vi "getLockStatus.vi"(8 "error":errorcluster, 11 "connection ID":refnum<k5>) -> (0 "error out":errorcluster, 1 "authorized":bool, 2 "locked":bool, 3 "connection ID out":refnum<k5>)   [LabVIEW 2016, in "sen_api.lvlib"]
doc: "This function returns if the device is locked and if the current client is authorized to use the device."
uses:
  sen_api.lvlib
panel:
  out "jsonRespIn":string
  out "JSON-response":string="{\"jsonrpc\":\"2.0\",\"method\":\"\",\"params\":[5,1.245,true,\"name\"],\"id\":\"1\"}"
  out "JSON request":string
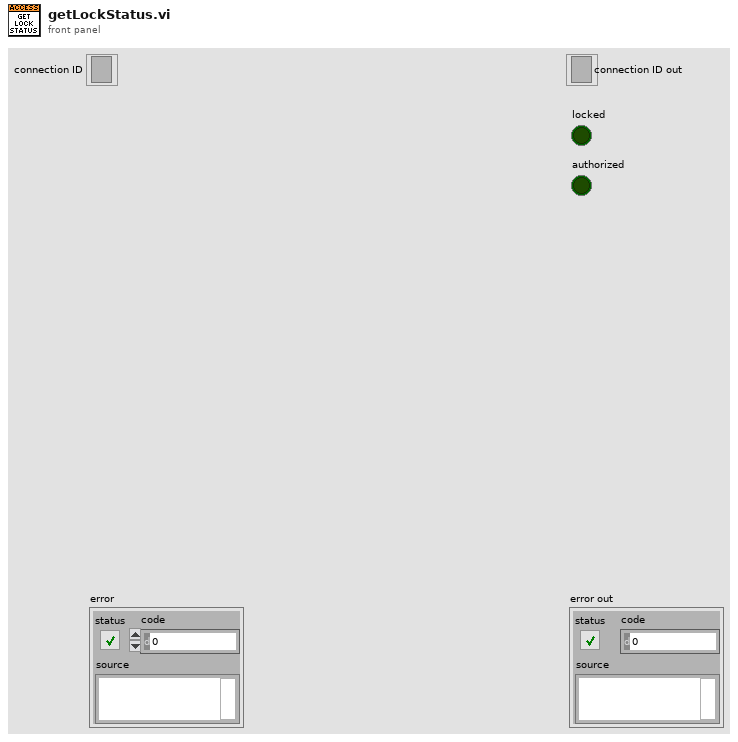
[diagram p1: front panel]
types:
  T1 = cluster{"jsonrpc":string, "method":string, "params":string[], "id":string, "api":i32, "pid":string}
  T2 = enum16{"Standard", "Buffered", "CRLF", "Immediate"}
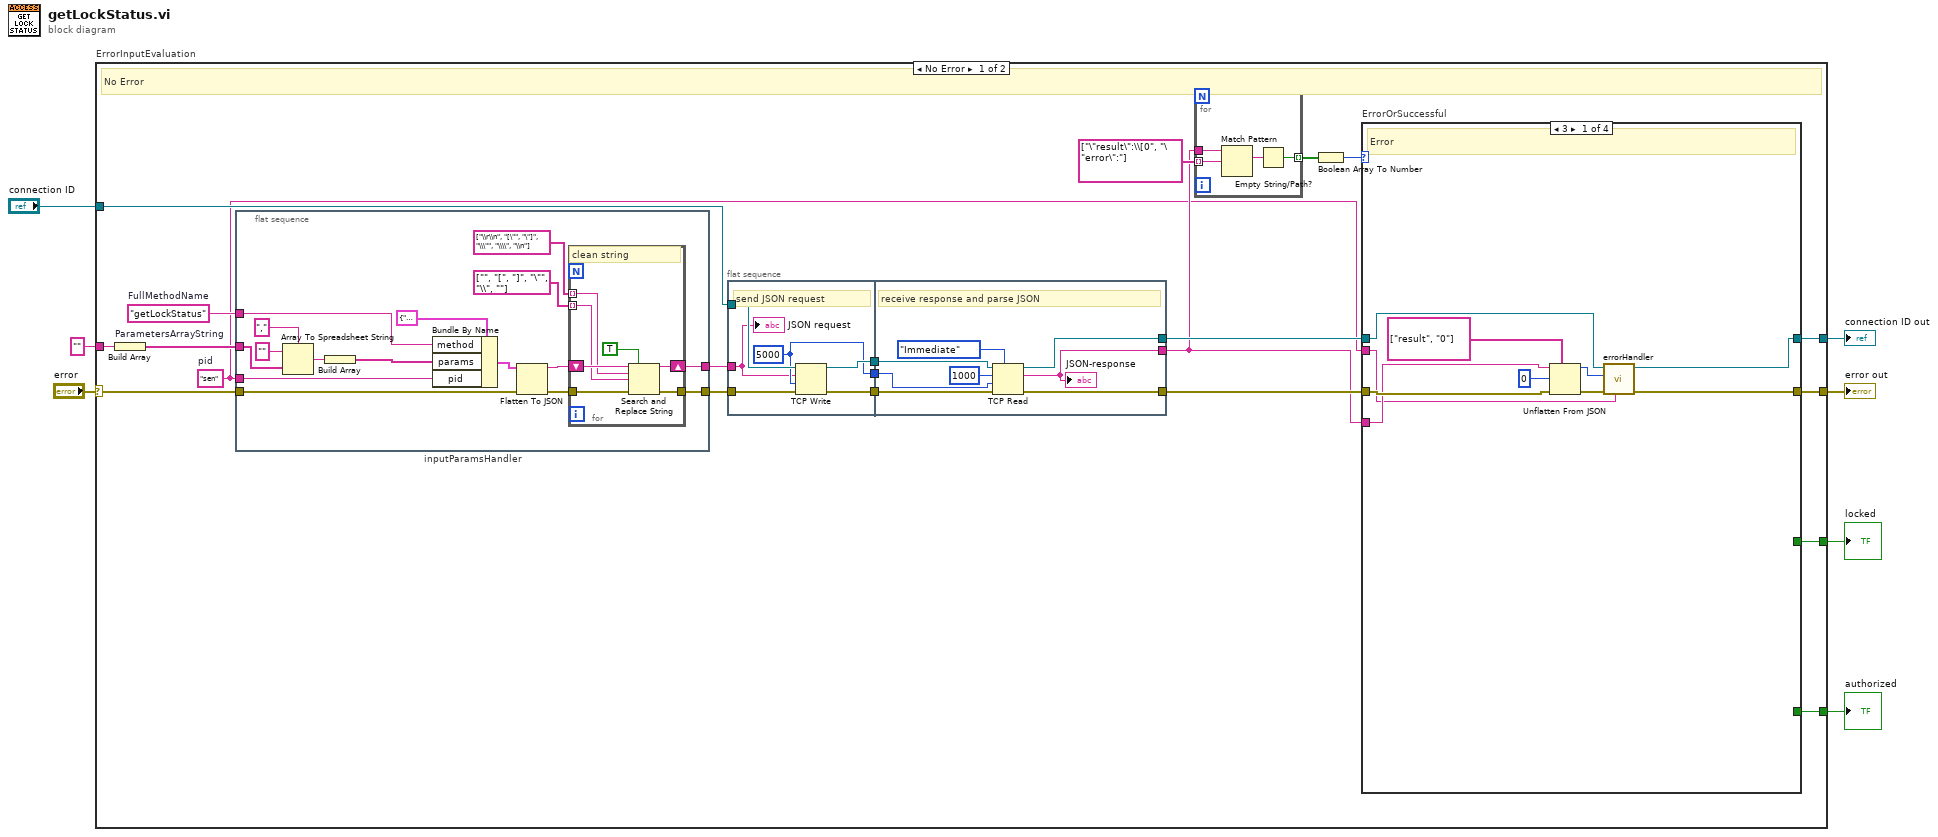
[diagram p0: block diagram]
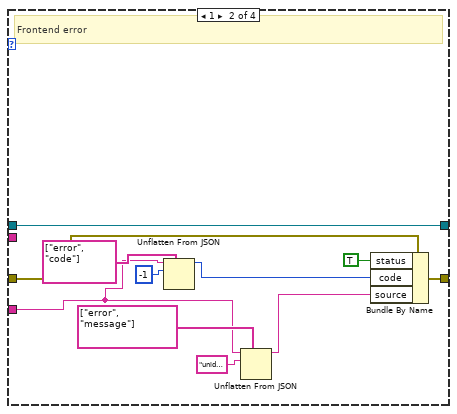
[diagram p2: hidden frame]
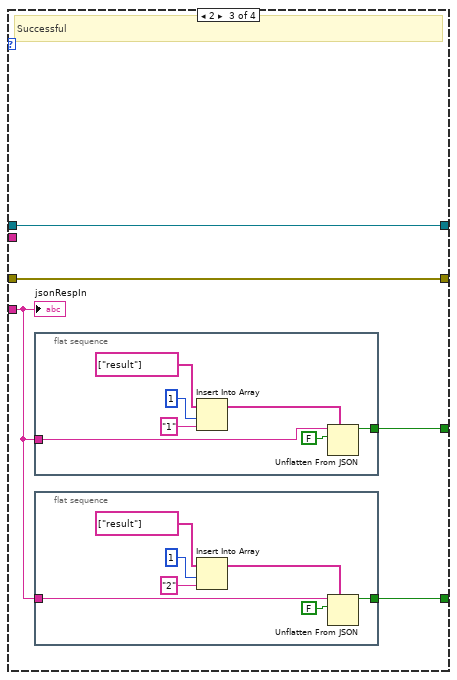
[diagram p3: hidden frame]
diagram:
  n1 = case "ErrorInputEvaluation" shown="No Error" "error" {
    selector: "error" -> [w15 w112]
    tunnel: "connection ID" -> [w25 w113]
    tunnel: [w17 w112] -> w6
    tunnel: [w18 w113] -> w5
    tunnel: "" -> [w10 _]
    tunnel: [w9 _] -> w2
    tunnel: [w8 _] -> w1
    frame No Error {
      w11 = "sen"  # pid
      w16 = "getLockStatus"  # FullMethodName
      # "No Error"
      n2 = Build Array "ParametersArrayString"(w10) -> (w14:string[])
      n3 = flat-sequence "inputParamsHandler" {
        tunnel: [w32] -> w13
        tunnel: w14 -> [w39]
        tunnel: w15 -> [w37]
        tunnel: [w34] -> w12
        tunnel: w16 -> [w40]
        tunnel: w11 -> [w29]
        frame #0 {
          n4 = Array To Spreadsheet String(delimiter (Tab)=",", array=w39, 3:"" ("format string")) -> (spreadsheet string=w42:string)
          n5 = Build Array "Build Array"(w42) -> (w38:string[])
          n6 = Bundle By Name(cluster=T1 {"jsonrpc"="2.0", "method"="com.attocube.amc.res.setRESReadOutFreq", "params"=[], "id"="1", "api"=2, "pid"=""}, "method"=w40, "params"=w38, "pid"=w29) -> (w41:T1)
          n7 = Flatten To JSON(anything=w41, error in (no error)=w37) -> (JSON string=w33:string, 11:w35:errorcluster)  [unwired: 1 in]
          n8 = for {
            tunnel: string[] ["\\r\\n", "[\"", "\"]", "\\\"", "\\\\", "\\n"] ("search string") -> [w48] mode=indexing
            tunnel: string[] ["", "[", "]", "\"", "\\", ""] ("replace string (\"\")") -> [w47] mode=indexing
            shift-right: [w50] -> w32
            shift-left: w33 -> [w49]
            tunnel: w35 -> [w46]
            tunnel: [w45] -> w34
            # "clean string"
            n9 = Search and Replace String(replace all?=TRUE ("replace all? (F)"), input string=w49, search string=w48, replace string=w47, error in=w46) -> (result string=w50:string, error out=w45:errorcluster)  [unwired: 3 in, 2 out]
          }
        }
      }
      n10 = flat-sequence {
        tunnel: w25 -> [w103]
        tunnel: [w101] -> w28
        tunnel: [w102] -> w27
        tunnel: w12 -> [w98]
        tunnel: [w100] -> w26
        tunnel: w13 -> [w99]
        tunnel: [w107] -> w21
        tunnel: w28 -> [w109]
        tunnel: w27 -> [w108]
        tunnel: [w105] -> w20
        tunnel: w26 -> [w106]
        tunnel: [w104] -> w19
        frame #0 {
          w100 = 5000 ("timeout ms (25000)")
          # "send JSON request"
          n11 = TCP Write(connection ID=w103, data in=w99, error in (no error)=w98, 9:w100) -> (connection ID out=w101:refnum<k5>, error out=w102:errorcluster)  [unwired: 1 out]
          "JSON request" <- w99
        }
        frame #1 {
          # "receive response and parse JSON"
          n12 = TCP Read(connection ID=w109, bytes to read=1000, error in (no error)=w108, 7:T2."Immediate" ("mode (standard)"), 9:w106) -> (connection ID out=w107:refnum<k5>, data out=w104:string, error out=w105:errorcluster)
          "JSON-response" <- w104
        }
      }
      n13 = for {
        tunnel: string[] ["\"result\":\\[0", "\"error\":"] ("path") -> [w54] mode=indexing
        tunnel: [w52] -> w23 mode=indexing
        tunnel: w19 -> [w55]
        n14 = Match Pattern(string=w55, regular expression=w54) -> (match substring=w53:string)  [unwired: 1 in, 3 out]
        n15 = Empty String/Path?(string/path=w53) -> (empty?=w52:bool)
      }
      n16 = Boolean Array To Number(Boolean array=w23) -> (number=w22:u32)
      n17 = case "ErrorOrSuccessful" shown="3" w22 {
        tunnel: w19 -> [w59 w68 w79 _]
        tunnel: w21 -> [w63 w66 w81 w97]
        tunnel: [w61 w66 w81 w97] -> w18
        tunnel: [w62 w69 w80 w96] -> w17
        tunnel: w20 -> [w65 w67 w80 w96]
        tunnel: w11 -> [w56 _ _ _]
        tunnel: [_ _ w78 _] -> w9
        tunnel: [_ _ w77 _] -> w8
        frame 3 {
          # "Error"
          n18 = Unflatten From JSON(path=string[] ["result", "0"], JSON string=w59, type and defaults=0, error in (no error)=w65) -> (value=w57:i32, error out=w64:errorcluster)  [unwired: 3 in]
          n19 = call "errorHandler.vi"("pid"=w56, "error in"=w64, "errNbr"=w57, "connection ID"=w63) -> ("error out 2"=w62:errorcluster, "connection ID out"=w61:refnum<k5>)  [unwired: 6 in]
        }
        frame 1 {
          # "Frontend error"
          n20 = Unflatten From JSON(path=string[] ["error", "code"], JSON string=w68, type and defaults=-1) -> (value=w75:i32)  [unwired: 4 in, 1 out]
          n21 = Unflatten From JSON(path=string[] ["error", "message"], JSON string=w68, type and defaults="unidentified error") -> (value=w76:string)  [unwired: 4 in, 1 out]
          n22 = Bundle By Name(cluster=w67, "status"=TRUE, "code"=w75, "source"=w76) -> (w69:errorcluster)
        }
        frame 2 {
          # "Successful"
          n23 = flat-sequence "out_bool" {
            tunnel: w79 -> [w94]
            tunnel: [w89] -> w78
            frame #0 {
              n24 = Insert Into Array "Insert Into Array"(array=string[] ["result"] ("path"), index=1, new element="1" ("idx")) -> (w91:string[])
              n25 = Unflatten From JSON(path=w91, JSON string=w94, type and defaults=FALSE) -> (value=w89:bool)  [unwired: 4 in, 1 out]
            }
          }
          n26 = flat-sequence "out_bool" {
            tunnel: w79 -> [w87]
            tunnel: [w82] -> w77
            frame #0 {
              n27 = Insert Into Array "Insert Into Array"(array=string[] ["result"] ("path"), index=1, new element="2" ("idx")) -> (w84:string[])
              n28 = Unflatten From JSON(path=w84, JSON string=w87, type and defaults=FALSE) -> (value=w82:bool)  [unwired: 4 in, 1 out]
            }
          }
          "jsonRespIn" <- w79
        }
        frame Default {
          # "NoResponse"
        }
      }
    }
    frame Error {
      # "Error"
    }
  }
  "error out" <- w6
  "connection ID out" <- w5
  "locked" <- w2
  "authorized" <- w1
